vi "PDE Flexible Element_Grid Points.vi"() -> (2 "Grid Points":cluster{"X":dbl, "Y":dbl}[](array[cluster]), 3 "Boundary Points":cluster{"X":dbl, "Y":dbl}[](array[cluster]))   [LabVIEW 2023]
doc: "Generate grid points for PDE Flexible Element.vi example."
uses:
  <vilib>/Analysis/1siggen.llb/Ramp Pattern by Samples.vi
  <vilib>/Analysis/NI_AALBase.lvlib
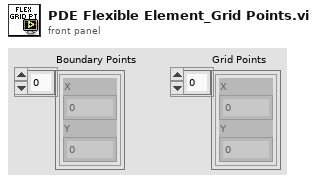
[diagram p1: front panel]
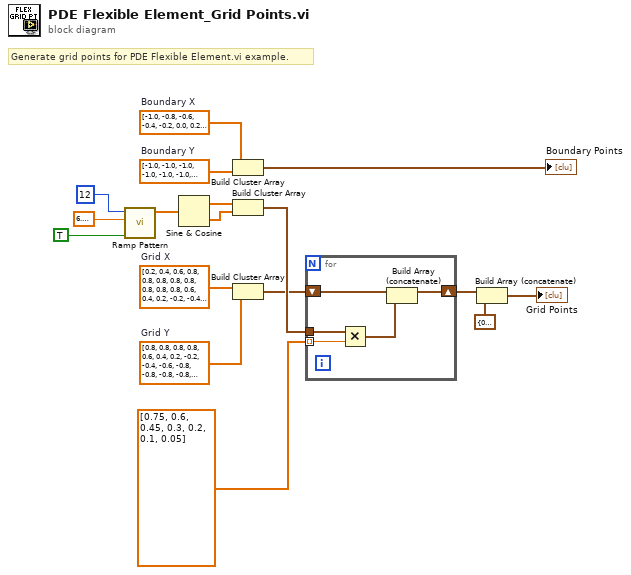
[diagram p0: block diagram]
diagram:
  w2 = dbl[] [0.8, 0.8, 0.8, 0.8, 0.6, 0.4, 0.2, -0.2, -0.4, -0.6, -0.8, -0.8, -0.8, -0.8, -0.8, -0.8, -0.8, -0.8, -0.6, -0.4, -0.2, 0.2, 0.4, 0.6, 0.8, 0.8, 0.8, 0.8, 0.6, -0.6, -0.6, 0.6]  # Grid Y
  w3 = dbl[] [0.2, 0.4, 0.6, 0.8, 0.8, 0.8, 0.8, 0.8, 0.8, 0.8, 0.8, 0.6, 0.4, 0.2, -0.2, -0.4, -0.6, -0.8, -0.8, -0.8, -0.8, -0.8, -0.8, -0.8, -0.8, -0.6, -0.4, -0.2, 0.6, 0.6, -0.6, -0.6]  # Grid X
  w6 = dbl[] [-1.0, -1.0, -1.0, -1.0, -1.0, -1.0, -1.0, -1.0, -1.0, -1.0, -1.0, -0.8, -0.6, -0.4, -0.2, 0.0, 0.2, 0.4, 0.6, 0.8, 1.0, 1.0, 1.0, 1.0, 1.0, 1.0, 1.0, 1.0, 1.0, 1.0, 1.0, 0.8, 0.6, 0.4, 0.2, 0.0, -0.2, -0.4, -0.6, -0.8]  # Boundary Y
  w7 = dbl[] [-1.0, -0.8, -0.6, -0.4, -0.2, 0.0, 0.2, 0.4, 0.6, 0.8, 1.0, 1.0, 1.0, 1.0, 1.0, 1.0, 1.0, 1.0, 1.0, 1.0, 1.0, 0.8, 0.6, 0.4, 0.2, 0.0, -0.2, -0.4, -0.6, -0.8, -1.0, -1.0, -1.0, -1.0, -1.0, -1.0, -1.0, -1.0, -1.0, -1.0]  # Boundary X
  # "Generate grid points for PDE Flexible Element.vi example."
  n1 = call-poly <vilib>:"Ramp Pattern.vi"("exclude end?"=TRUE, "end"=6.283185307179586, "samples"=12) -> ("Ramp Pattern"=w17:dbl[])  [unwired: 7 in, 1 out]
  n2 = Sine & Cosine(0:w17) -> (1:w13:dbl[], 2:w1:dbl[])
  n3 = Build Cluster Array(w7, w6) -> (→"Boundary Points":cluster{"Numeric":dbl, "Numeric":dbl}[])
  n4 = Build Cluster Array(w13, w1) -> (w12:cluster{dbl, dbl}[])
  n5 = Build Cluster Array(w3, w2) -> (w4:cluster{"Numeric":dbl, "Numeric":dbl}[])
  n6 = for {
    shift-right: [w20] -> w9
    shift-left: w4 -> [w21]
    tunnel: w12 -> [w22]
    tunnel: dbl[] [0.75, 0.6, 0.45, 0.3, 0.2, 0.1, 0.05] ("reversed array") -> [w18] mode=indexing
    n7 = Multiply(x=w22, y=w18) -> (x*y=w19:cluster{dbl, dbl}[])
    n8 = Build Array (concatenate)(w21, w19) -> (w20:cluster{"Numeric":dbl, "Numeric":dbl}[])
  }
  n9 = Build Array (concatenate)(w9, cluster{"X":dbl, "Y":dbl} {"X"=0.0, "Y"=0.0} ("point")) -> (→"Grid Points":cluster{"X":dbl, "Y":dbl}[])
